vi "sincos.vi"() -> ()   [LabVIEW 2015]
uses:
  <vilib>/rvi/FXPMathLib/FxpSinAndCos/subVIs/nifxpmath_SinAndCos_SimConfig.ctl
  <vilib>/Analysis/baseanly.llb/Mean (DBL).vi
  <vilib>/rvi/FXPMathLib/FxpSinAndCos/simVIs/DllFxpSinAndCosTemp_sub.vi
  <vilib>/rvi/FXPMathLib/FxpSinAndCos/XNode/nifxpmath_SinAndCos.xnode
  <vilib>/Analysis/NI_AALBase.lvlib
panel:
  out "sinsgl_stddev":dbl format="%0.5f"
  out "sinsgl_stddev":dbl format="%0.5f"
  out "sinfxp_stddev":dbl format="%0.5f"
  out "sinfxp_stddev":dbl format="%0.5f"
  out "cosfxp_mean":dbl format="%0.5f"
  out "sinfxp_mean":dbl format="%0.5f"
  out "cosfxp_max":dbl
  out "sinfxp_max":dbl
  out "stdcosfxp_mean":dbl format="%0.2f"
  out "stdsinfxp_mean":dbl format="%0.2f"
  out "stdcosfxp_max":dbl
  out "stdsinfxp_max":dbl
  out "cossgl_mean":dbl format="%0.5f"
  out "sinsgl_mean":dbl format="%0.5f"
  out "cossgl max":dbl
  out "sinsgl_max":dbl
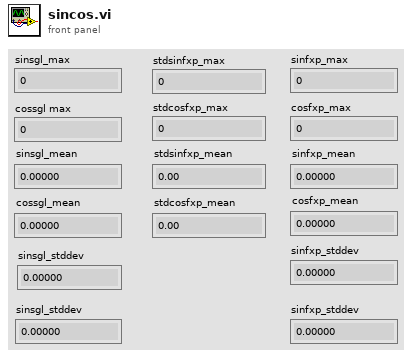
[diagram p1: front panel]
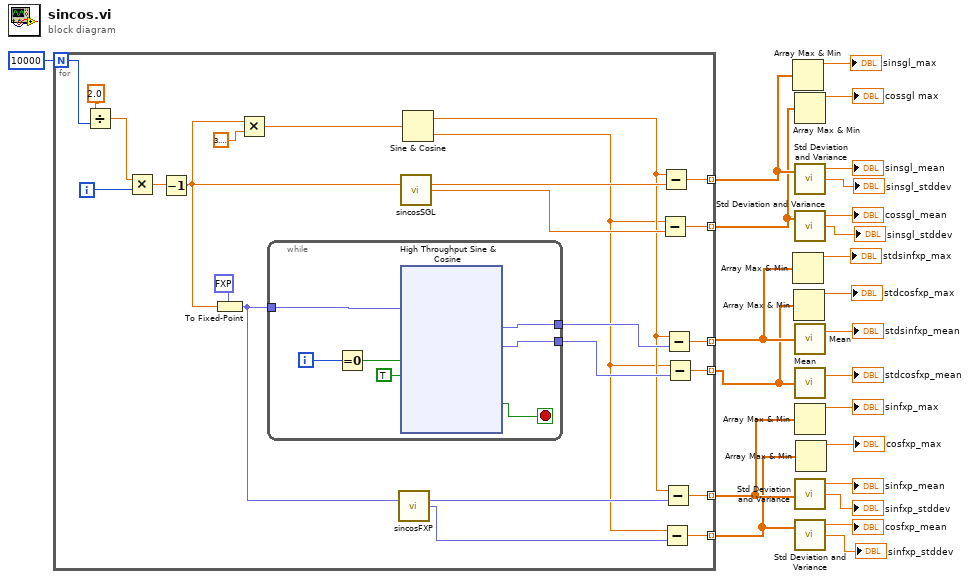
[diagram p0: block diagram]
diagram:
  n1 = for {
    N: 10000 -> [w28]
    tunnel: [w37] -> w22 mode=indexing
    tunnel: [w36] -> w21 mode=indexing
    tunnel: [w35] -> w20 mode=indexing
    tunnel: [w34] -> w19 mode=indexing
    tunnel: [w33] -> w18 mode=indexing
    tunnel: [w32] -> w17 mode=indexing
    i -> [w26]
    n2 = Divide(x=2.0 ("y"), y=w28) -> (x/y=w27:dbl)
    n3 = Multiply(x=w27, y=w26) -> (x*y=w25:dbl)
    n4 = Decrement(x=w25) -> (x-1=w24:dbl)
    n5 = To Fixed-Point(fixed-point type=fxp<+/-,16,1> 0.0 ("x (pi)"), number=w24) -> (fixed-point=w46:fxp<+/-,16,1>)
    n6 = Multiply(x=w24, y=3.141592653589793) -> (x*y=w31:dbl)
    n7 = while {
      tunnel: w46 -> [w54]
      tunnel: [w49] -> w42
      tunnel: [w48] -> w43
      i -> [w53]
      stop <- w50 stop-if-true
      n8 = Equal To 0?(x=w53) -> (x = 0?=w52:bool)
      n9 = xnode "High Throughput Sine & Cosine"("x (pi)"=w54, "input valid"=w52, "ready for output (T)"=TRUE) -> ("sin(x)"=w49:fxp<+/-,16,2>, "cos(x)"=w48:fxp<+/-,16,2>, "output valid"=w50:bool)  [unwired: 1 out]
    }
    n10 = call "sincosFXP.vi"("x"=w46) -> ("sinx"=w40:fxp<+/-,16,2>, "cosx"=w38:fxp<+/-,16,2>)  [unwired: 13 in]
    n11 = call "sincosSGL.vi"("x"=w24) -> ("sinx"=w45:sgl, "cosx"=w44:sgl)  [unwired: 13 in]
    n12 = Sine & Cosine(0:w31) -> (1:w41:dbl, 2:w39:dbl)
    n13 = Subtract(x=w39, y=w44) -> (x-y=w36:dbl)
    n14 = Subtract(x=w41, y=w45) -> (x-y=w37:dbl)
    n15 = Subtract(x=w39, y=w38) -> (x-y=w32:dbl)
    n16 = Subtract(x=w41, y=w40) -> (x-y=w33:dbl)
    n17 = Subtract(x=w41, y=w42) -> (x-y=w35:dbl)
    n18 = Subtract(x=w39, y=w43) -> (x-y=w34:dbl)
  }
  n19 = Array Max & Min(array=w22) -> (max value=→"sinsgl_max":dbl)  [unwired: 3 out]
  n20 = Array Max & Min(array=w20) -> (max value=→"stdsinfxp_max":dbl)  [unwired: 3 out]
  n21 = Array Max & Min(array=w19) -> (max value=→"stdcosfxp_max":dbl)  [unwired: 3 out]
  n22 = Array Max & Min(array=w21) -> (max value=→"cossgl max":dbl)  [unwired: 3 out]
  n23 = call <vilib>:"Std Deviation and Variance.vi"("X"=w22) -> ("mean"=→"sinsgl_mean":dbl, "standard deviation"=→"sinsgl_stddev":dbl)  [unwired: 1 in, 1 out]
  n24 = call <vilib>:"Std Deviation and Variance.vi"("X"=w21) -> ("mean"=→"cossgl_mean":dbl, "standard deviation"=→"sinsgl_stddev":dbl)  [unwired: 1 in, 1 out]
  n25 = call-poly <vilib>:"Mean.vi"("X"=w20) -> ("mean"=→"stdsinfxp_mean":dbl)  [unwired: 1 out]
  n26 = call-poly <vilib>:"Mean.vi"("X"=w19) -> ("mean"=→"stdcosfxp_mean":dbl)  [unwired: 1 out]
  n27 = Array Max & Min(array=w18) -> (max value=→"sinfxp_max":dbl)  [unwired: 3 out]
  n28 = call <vilib>:"Std Deviation and Variance.vi"("X"=w18) -> ("mean"=→"sinfxp_mean":dbl, "standard deviation"=→"sinfxp_stddev":dbl)  [unwired: 1 in, 1 out]
  n29 = call <vilib>:"Std Deviation and Variance.vi"("X"=w17) -> ("mean"=→"cosfxp_mean":dbl, "standard deviation"=→"sinfxp_stddev":dbl)  [unwired: 1 in, 1 out]
  n30 = Array Max & Min(array=w17) -> (max value=→"cosfxp_max":dbl)  [unwired: 3 out]
